vi "全场定位模块.vi"(0 "VISA resource name":refnum<visa-resource-name>="ASRL4::INSTR" caption="VISA资源名称") -> (3 "VISA资源名称输出":refnum<visa-resource-name>, 4 "y":sgl format="%_6f", 6 "x":sgl format="%_6f", 8 "Zangle":sgl format="%_6f", 10 "pd":bool, 14 "错误输出2":errorcluster, 15 "缓冲区监视器":string)   [LabVIEW 2016]
uses:
  <vilib>/Instr/_visa.llb/VISA Configure Serial Port (Instr).vi
  <vilib>/imath/engines/lvmath2/RunTimeEngine/Managers/WorkSpace/UID Generator.vi
  <vilib>/imath/engines/lvmath2/RunTimeEngine/BuiltInFunctions/is_empty/NIMS_is_empty(GV).vi
  <instcachedir>/0/NIMS_is_empty(GV)_FC7E7C3D9544432CB6AA2416ADCF6D56.lvgen/NIMS_is_empty(GV)_FC7E7C3D9544432CB6AA2416ADCF6D56_000.vi
  <vilib>/imath/engines/lvmath2/RunTimeEngine/BuiltInFunctions/length/NIMS_length(GV).vi
  <instcachedir>/0/NIMS_length(GV)_08A3D13377FD4E4B96F5795FBF3698FA.lvgen/NIMS_length(GV)_08A3D13377FD4E4B96F5795FBF3698FA_003.vi
  <vilib>/imath/engines/lvmath2/RunTimeEngine/RunTimeType/NIMS_RunTimeType_From StrictType (excl LVString).vi
  <instcachedir>/0/NIMS_RunTimeType_From StrictType (excl LVString)_BBF44FB49F834B71AF7A14CCEDF8BECD.lvgen/NIMS_RunTimeType_From StrictType (excl LVString)_BBF44FB49F834B71AF7A14CCEDF8BECD_000.vi
  <vilib>/imath/engines/lvmath2/RunTimeEngine/LocalVariableDefStatement/MC_LocalVariableDefStatement_Display.vi
  <vilib>/imath/engines/lvmath2/RunTimeEngine/RangeToken/NIMS_Range_R3 - Integer.vi
  <instcachedir>/0/NIMS_Range_R3 - Integer_A435E2FF893B4C718FD5055FE39FE2F6.lvgen/NIMS_Range_R3 - Integer_A435E2FF893B4C718FD5055FE39FE2F6_000.vi
  <vilib>/imath/engines/lvmath2/RunTimeEngine/CommandStatement/MC_CommandStatement_break.vi
  <vilib>/imath/engines/lvmath2/RunTimeEngine/IndexRead/NIMS M(S,S).vi
  <instcachedir>/0/NIMS M(S,S)_AC51E74150A542F7991B9634C66F3096.lvgen/NIMS M(S,S)_AC51E74150A542F7991B9634C66F3096_003.vi
  <vilib>/imathl/engines/lvmath/Functions/Error Handling/Create Error.vi
  <vilib>/imath/engines/lvmath2/RunTimeEngine/VariableToken/NIMS_VariableToken_CondDefinedDefinedByReplace.vi
  <instcachedir>/0/NIMS_VariableToken_CondDefinedDefinedByReplace_D162CFFC24174562A9FEA619A91E1A56.lvgen/NIMS_VariableToken_CondDefinedDefinedByReplace_D162CFFC24174562A9FEA619A91E1A56_003.vi
  <vilib>/imath/engines/lvmath2/RunTimeEngine/VariableToken/NIMS_VariableToken_CondDefined.vi
  <instcachedir>/0/NIMS_VariableToken_CondDefined_06E9DA95BD4D46A6BA55EC651A891960.lvgen/NIMS_VariableToken_CondDefined_06E9DA95BD4D46A6BA55EC651A891960_005.vi
  <vilib>/imath/engines/lvmath2/RunTimeEngine/IndexReplace/NIMS M(S,S)=S.vi
  <instcachedir>/0/NIMS M(S,S)=S_98E40400474E4398B113AE20298B4F82.lvgen/NIMS M(S,S)=S_98E40400474E4398B113AE20298B4F82_003.vi
  <vilib>/imath/engines/lvmath2/RunTimeEngine/ErrorHandling/NIMS_Create Error From Enums.vi
  <instcachedir>/0/NIMS_VariableToken_CondDefined_06E9DA95BD4D46A6BA55EC651A891960.lvgen/NIMS_VariableToken_CondDefined_06E9DA95BD4D46A6BA55EC651A891960_006.vi
  <vilib>/imath/engines/lvmath/Functions/Error Handling/MergeErrorsWrapper.vi
  <vilib>/imath/engines/lvmath2/RunTimeEngine/Managers/SymbolTable/Clear UID.vi
  <vilib>/imath/engines/lvmath2/RunTimeEngine/NodeEndStatement/NIMS_NodeEndStatement_Output.vi
  <instcachedir>/0/NIMS_NodeEndStatement_Output_53EC0D466D134D7ABD903AC30B43404B.lvgen/NIMS_NodeEndStatement_Output_53EC0D466D134D7ABD903AC30B43404B_013.vi
  <instcachedir>/0/NIMS_NodeEndStatement_Output_53EC0D466D134D7ABD903AC30B43404B.lvgen/NIMS_NodeEndStatement_Output_53EC0D466D134D7ABD903AC30B43404B_011.vi
  <vilib>/imath/engines/lvmath2/RunTimeEngine/ErrorHandling/NIMS_Finalize Error.vi
  <vilib>/imath/engines/lvmath2/RunTimeEngine/BuiltInFunctions/is_empty/NIMS_is_empty(GM).vi
  <instcachedir>/0/NIMS_is_empty(GM)_AF8F13F4B7FD436CB1855477E2504B8A.lvgen/NIMS_is_empty(GM)_AF8F13F4B7FD436CB1855477E2504B8A_005.vi
  <vilib>/imath/engines/lvmath2/RunTimeEngine/NodeEndStatement/NIMS_NodeEndStatement_Get Vector.vi
  <instcachedir>/0/NIMS_NodeEndStatement_Get Vector_9E4547DF38A84F62A7E036B4CE3D251C.lvgen/NIMS_NodeEndStatement_Get Vector_9E4547DF38A84F62A7E036B4CE3D251C_002.vi
  <instcachedir>/0/NIMS_NodeEndStatement_Output_53EC0D466D134D7ABD903AC30B43404B.lvgen/NIMS_NodeEndStatement_Output_53EC0D466D134D7ABD903AC30B43404B_004.vi
  <instcachedir>/0/NIMS_NodeEndStatement_Output_53EC0D466D134D7ABD903AC30B43404B.lvgen/NIMS_NodeEndStatement_Output_53EC0D466D134D7ABD903AC30B43404B_010.vi
  <vilib>/imath/engines/lvmath2/RunTimeEngine/Managers/SymbolTable/NIMS_WorkSpace.lvlib
panel:
  out "字节缓冲区长度":i32
  out "错误输出1":errorcluster
  in  "串口设置":T1={"波特率"=115200, "数据位"=8, "校验"=enum."None", "停止位"=10, "流控制"=0} {"流控制" items=["无"=0, "XON/XOFF"=1, "RTS/CTS"=2, "DTR/DSR"=4]; "停止位" items=["1.0"=10, "1.5"=15, "2.0"=20]; "数据位" min=5 max=8 step=1; "波特率" items=["115200"=115200, "460800"=460800, "75"=75, "110"=110, "134"=134, "150"=150, "300"=300, "600"=600, "1200"=1200, "1800"=1800, "2400"=2400, "4800"=4800, "7200"=7200, "9600"=9600, "14400"=14400, "19200"=19200, "28800"=28800, "38400"=38400, "56000"=56000, "57600"=57600, "128000"=128000, "230400"=230400]}
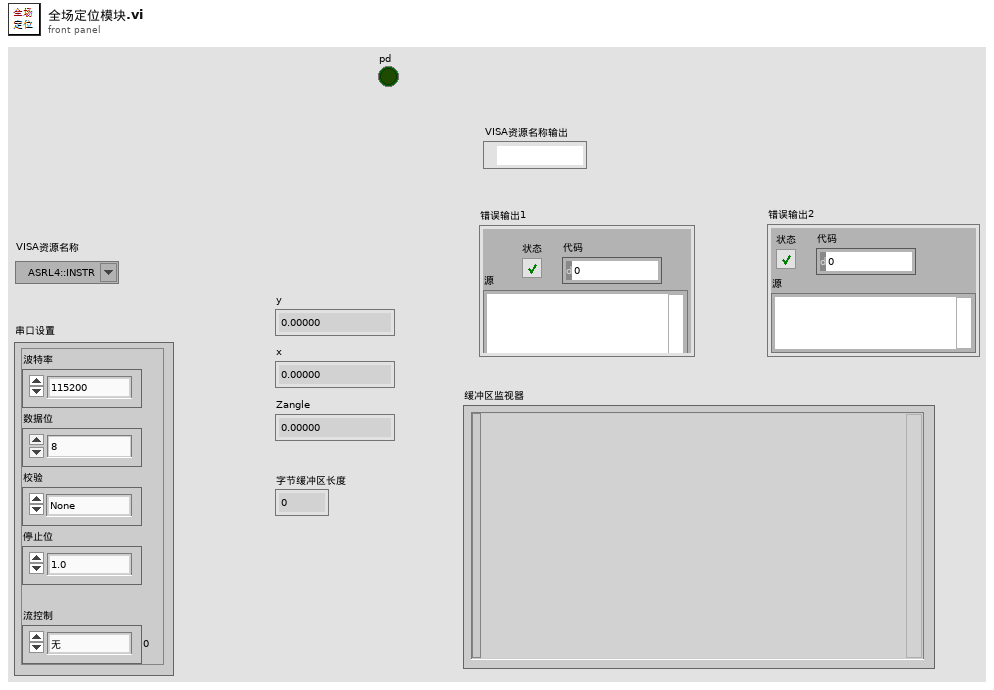
[diagram p1: front panel]
types:
  T1 = cluster{"波特率":u32, "数据位":u16, "校验":enum16{"None", "Odd", "Even", "Mark", "Space"}, "停止位":u16, "流控制":u16}
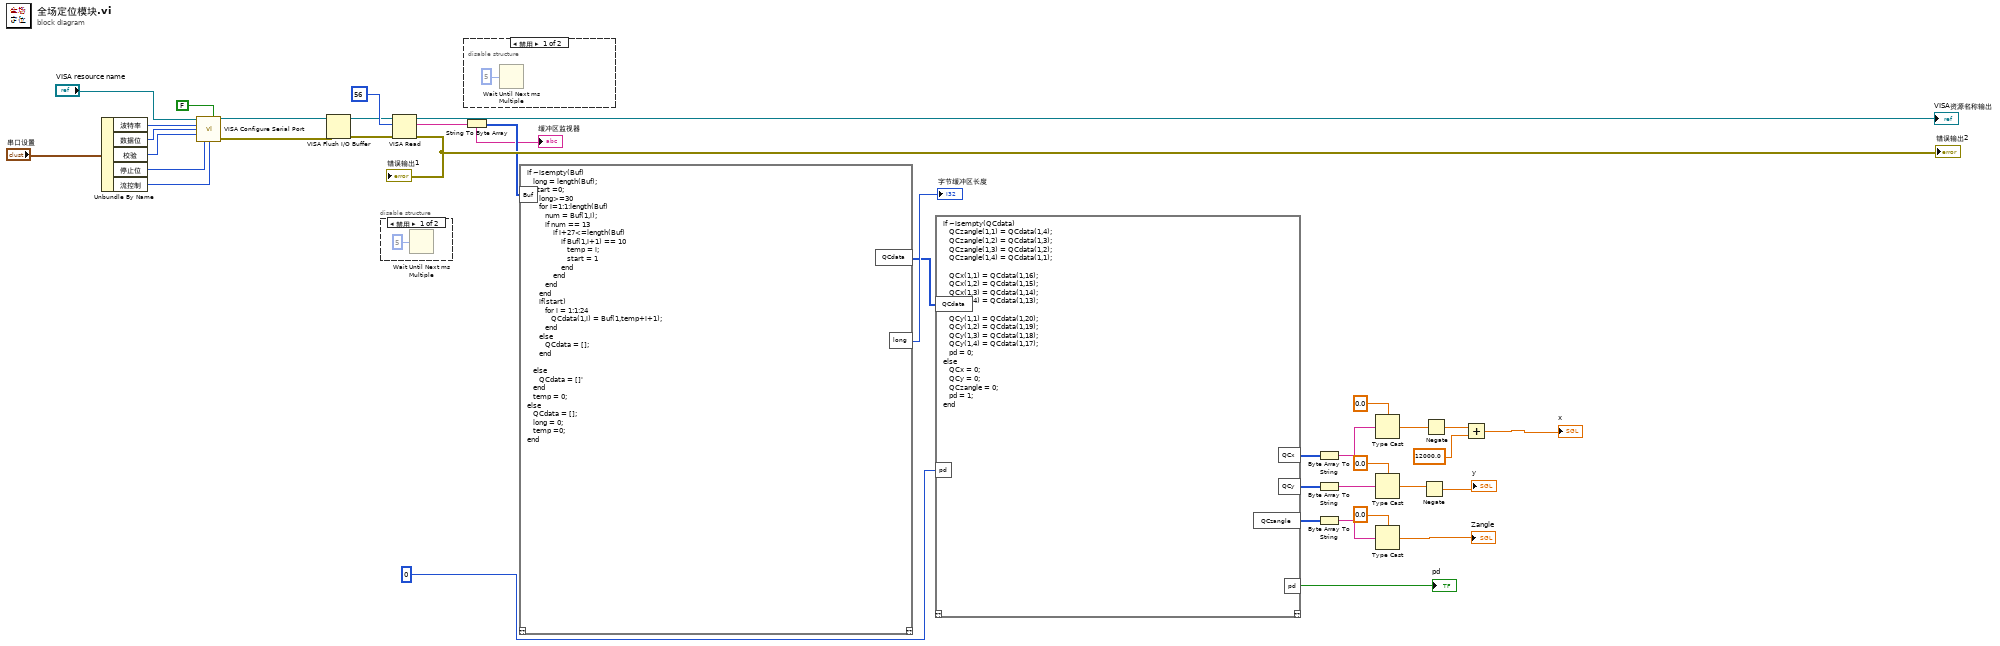
[diagram p0: block diagram]
diagram:
  n1 = Unbundle By Name("串口设置") -> ("波特率"=w35:u32, "数据位"=w34:u16, "校验"=w33:enum16{"None", "Odd", "Even", "Mark", "Space"}, "停止位"=w32:u16, "流控制"=w30:u16)
  n2 = call-poly "VISA Configure Serial Port"("VISA resource name"="VISA resource name", "Enable Termination\nChar (T)"=FALSE ("Enable Termination\nChar (T)"), "baud rate (9600)"=w35, "data bits (8)"=w34, "parity (0:none)"=w33, "stop bits (10: 1 bit)"=w32, "flow control (0:none)"=w30) -> ("VISA resource name out"=w27:refnum<visa-resource-name>, "error out"=w26:errorcluster)  [unwired: 2 in, 5 out]
  n3 = VISA Flush I/O Buffer(VISA resource name=w27, error in (no error)=w26) -> (VISA resource name out=w13:refnum<visa-resource-name>, error out=w14:errorcluster)  [unwired: 1 in]
  n4 = disable-structure shown="禁用" {
    frame Disabled {
      n5 = Wait Until Next ms Multiple(millisecond multiple=u32 5 ("毫秒倍数")) -> ()  [unwired: 1 out]
    }
    frame Enabled {
    }
  }
  n6 = VISA Read(VISA resource name=w13, byte count=56, error in (no error)=w14) -> (VISA resource name out=→"VISA资源名称输出":refnum<visa-resource-name>, read buffer=w10:string, error out=→"错误输出1" →"错误输出2":errorcluster)  [unwired: 1 out]
  "缓冲区监视器" <- w10
  n7 = disable-structure shown="禁用" {
    frame Disabled {
      n8 = Wait Until Next ms Multiple(millisecond multiple=u32 5 ("毫秒倍数")) -> ()  [unwired: 1 out]
    }
    frame Enabled {
    }
  }
  n9 = String To Byte Array(string=w10) -> (unsigned byte array=w25:u8[])
  n10 = mathscript code="if ~isempty(Buf)\n   long = length(Buf);\n   start =0;\n   if long>=30\n      for i=1:1:length(Buf)\n         num = Buf(1,i);\n         if num == 13\n             if i+27<=length(Buf)\n                 if Buf(1,i+1) == 10  \n                    temp = i;\n                    start = 1\n                 end\n             end\n         end\n      end\n      if(start)\n         for i = 1:1:24\n            QCdata(1,i) = Buf(1,temp+i+1);\n         end\n      else\n         QCdata = [];\n      end\n     \n   else \n      QCdata = []'\n   end\n   temp = 0;\nelse\n   QCdata = [];\n   long = 0;\n   temp =0;\nend"("Buf"=w25) -> ("long"=→"字节缓冲区长度":i32, "QCdata"=w11:u8[][])  [unwired: 1 in, 1 out]
  n11 = mathscript code="if ~isempty(QCdata)\n   QCzangle(1,1) = QCdata(1,4);\n   QCzangle(1,2) = QCdata(1,3);\n   QCzangle(1,3) = QCdata(1,2);\n   QCzangle(1,4) = QCdata(1,1);\n\n   QCx(1,1) = QCdata(1,16);\n   QCx(1,2) = QCdata(1,15);\n   QCx(1,3) = QCdata(1,14);\n   QCx(1,4) = QCdata(1,13);\n\n   QCy(1,1) = QCdata(1,20);\n   QCy(1,2) = QCdata(1,19);\n   QCy(1,3) = QCdata(1,18);\n   QCy(1,4) = QCdata(1,17);\n   pd = 0;\nelse \n   QCx = 0;\n   QCy = 0;\n   QCzangle = 0;\n   pd = 1;\nend"("QCdata"=w11, "pd"=0) -> ("QCx"=w17:i32[], "QCy"=w12:i32[], "QCzangle"=w16:i32[], "pd"=→"pd":bool)  [unwired: 1 in, 1 out]
  n12 = Byte Array To String(unsigned byte array=w17) -> (string=w22:string)
  n13 = Byte Array To String(unsigned byte array=w12) -> (string=w20:string)
  n14 = Byte Array To String(unsigned byte array=w16) -> (string=w18:string)
  n15 = Type Cast(type=sgl 0.0, x=w22) -> (*(type *) &x=w4:sgl)
  n16 = Type Cast(type=sgl 0.0, x=w20) -> (*(type *) &x=w6:sgl)
  n17 = Type Cast(type=sgl 0.0, x=w18) -> (*(type *) &x=→"Zangle":sgl)
  n18 = Negate(x=w6) -> (-x=→"y":sgl)
  n19 = Negate(x=w4) -> (-x=w3:sgl)
  n20 = Add(x=w3, y=sgl 12000.0) -> (x+y=→"x":sgl)
